vi "Write Plugin Error.vi"(8 "error in (no error)":errorcluster, 9 "timeout in ms (0)":i32 format="%d ms", 10 "error":errorcluster, 11 "Plugin Interface in":refnum<class "Plugin Interface.lvclass">) -> (0 "error out":errorcluster, 3 "Plugin Interface out":refnum<class "Plugin Interface.lvclass">)   [LabVIEW 2017, in "DSF Core.lvlib" / "Plugin Interface.lvclass"]
uses:
  Plugin Interface.lvclass
  C:/Users/Admin/Desktop/Data Sharing Framework/Source/Core/Engine/Classes/Interfaces/Interface/Interface.lvclass
  Interface/Interface.lvclass/Interface.ctl
  Interface/Write Error Queue.vi
  Dispatcher/Error Timeout.vi
  Interface/Interface.lvclass
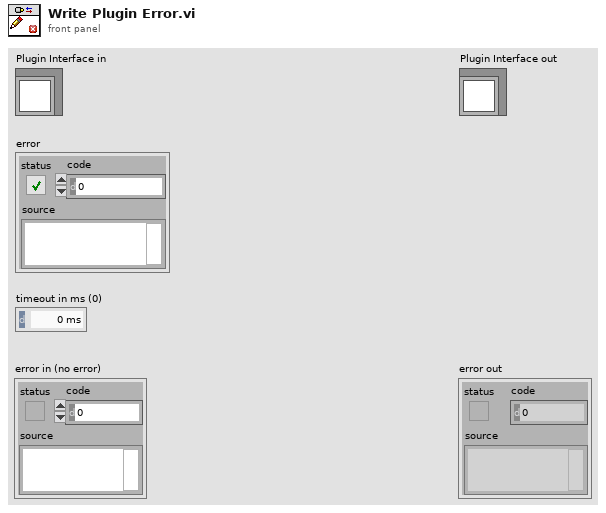
[diagram p1: front panel]
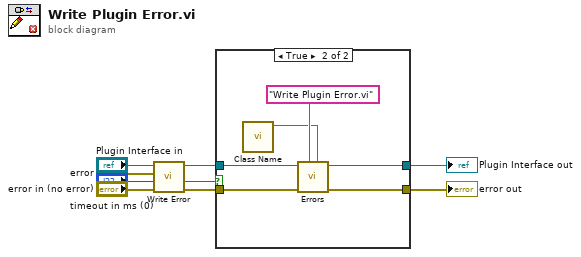
[diagram p0: block diagram]
diagram:
  n1 = call "Write Error.vi"("error in (no error)"="error in (no error)", "timeout in ms (0)"="timeout in ms (0)", "error"="error", "Interface in"="Plugin Interface in") -> ("error out"=w4:errorcluster, "timed out?"=w1:bool, "Interface out"=w5:refnum<class "Plugin Interface.lvclass">)  [unwired: 5 in]
  n2 = case shown="True" w1 {
    tunnel: w4 -> [w10 w15]
    tunnel: w5 -> [w11 w16]
    tunnel: [w11 w14] -> w3
    tunnel: [w10 w13] -> w2
    frame False {
    }
    frame True {
      n3 = call "Class Name.vi"() -> ("class name"=w12:string)  [unwired: 11 in]
      n4 = call-poly "Errors.vi"("error source class name"=w12, "error source vi name"="Write Plugin Error.vi", "error in (no error)"=w15, "Interface in"=w16) -> ("error out"=w13:errorcluster, "Interface out"=w14:refnum<class "Plugin Interface.lvclass">)  [unwired: 6 in]
    }
  }
  "error out" <- w2
  "Plugin Interface out" <- w3
